vi "3-1.vi"() -> ()   [LabVIEW 2022 SP3, in "AoC22.lvlib"]
uses:
  AoC22.lvlib
  5f5b93ce-2920-4ca0-a169-f55fba87441a.vi
  <vilib>/IlluminatedG/lv-stream/Stream.lvlib
panel:
  out "sum":i32
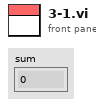
[diagram p1: front panel]
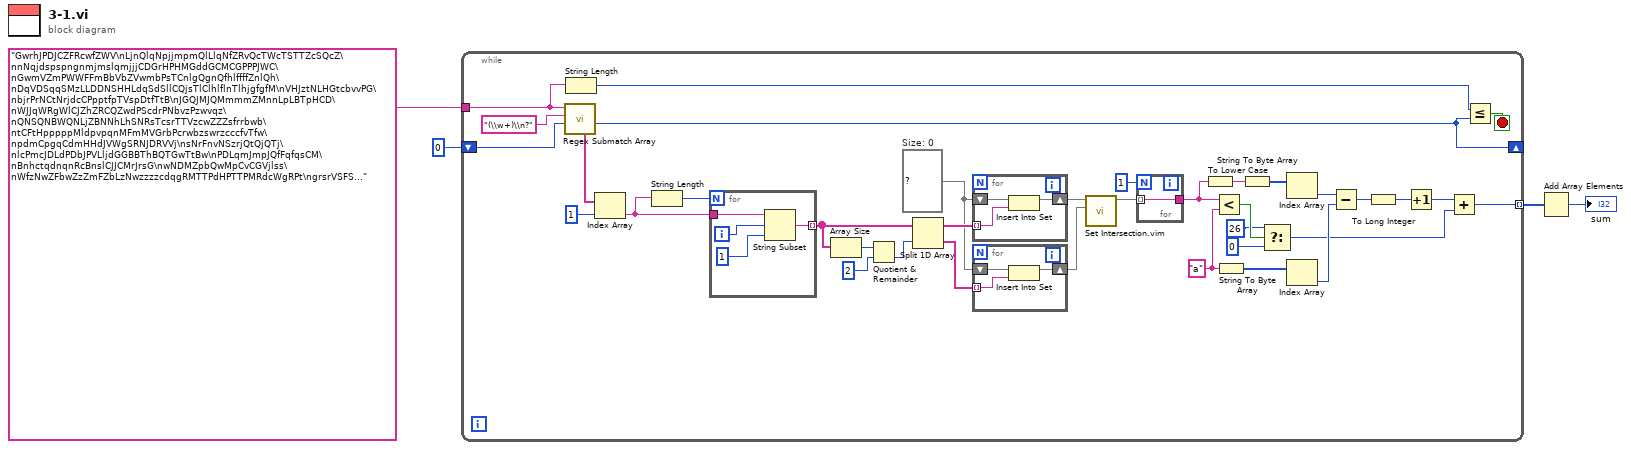
[diagram p0: block diagram]
diagram:
  n1 = while {
    tunnel: "GwrhJPDJCZFRcwfZWV\nLjnQlqNpjjmpmQlLlqNfZRvQcTWcTSTTZcSQcZ\nnNqjdspspngnmjmslqmjjjCDGrHPHMGddGCMCGPPPJWC\nGwmVZmPWWFFmBbVbZVwmbPsTCnlgQgnQfhlffffZnlQh\nDqVDSqqSMzLLDDNSHHLdqSdSllCQjsTlClhlflnTlhjgfgfM\nVHJztNLHGtcbvvPG\nbjrPrNCtNrjdcCPpptfpTVspDtfTtB\nJGQJMJQMmmmZMnnLpLBTpHCD\nWJJqWRgWlCJZhZRCQZwdPScdrPNbvzPzwvqz\nQNSQNBWQNLjZBNNhLhSNRsTcsrTTVzcwZZZsfrrbwb\ntCFtHpppppMldpvpqnMFmMVGrbPcrwbzswrzcccfvTfw\npdmCpgqCdmHHdJVWgSRNJDRVVj\nsNrFnvNSzrjQtQjQTj\nlcPmcJDLdPDbJPVLljdGGBBThBQTGwTtBw\nPDLqmJmpJQfFqfqsCM\nBnhctqdnqnRcBnslCJJCMrJrsG\nwNDMZpbQwMpCvCGVjlss\nWfzNwZFbwZzZmFZbLzNwzzzzcdqgRMTTPdHPTTPMRdcWgRPt\ngrsrVSFS..." -> [w8]
    shift-right: [w6] -> _
    shift-left: 0 -> [w39]
    tunnel: [w12] -> w2 mode=indexing
    stop <- w5 stop-if-true
    w25 = "a" ("y")
    w31 = set{string} {}  # Size: 0
    n2 = call <vilib>:"Regex Submatch Array.vi"("offset (0)"=w39, "regular expression"="(\\w+)\\n?", "string"=w8) -> ("offset past match"=w6:i32, "matches"=w38:string[])  [unwired: 6 in, 1 out]
    n3 = String Length(string=w8) -> (length=w7:i32)
    n4 = Index Array(array=w38, index=1) -> (element=w11:string)
    n5 = String Length(string=w11) -> (length=w10:i32)
    n6 = for {
      N: w10 -> [_]
      tunnel: w11 -> [w51]
      tunnel: [w48] -> w34 mode=indexing
      i -> [w50]
      n7 = String Subset(string=w51, offset (0)=w50, length (rest)=1 ("length (rest)")) -> (substring=w48:string)
    }
    n8 = Array Size(array=w34) -> (size(s)=w36:i32)
    n9 = Quotient & Remainder(x=w36, y=2) -> (floor(x/y)=w33:i32)  [unwired: 1 out]
    n10 = Split 1D Array(array=w34, index=w33) -> (first subarray=w32:string[], second subarray=w30:string[])
    n11 = for {
      tunnel: w32 -> [w46] mode=indexing
      shift-right: [w45] -> w29
      shift-left: w31 -> [w47]
      n12 = Insert Into Set(10:w46, 11:w47) -> (3:w45:set{string})  [unwired: 1 out]
    }
    n13 = for {
      tunnel: w30 -> [w43] mode=indexing
      shift-right: [w42] -> w28
      shift-left: w31 -> [w44]
      n14 = Insert Into Set(10:w43, 11:w44) -> (3:w42:set{string})  [unwired: 1 out]
    }
    n15 = call "Set Intersection.vim"("set 2"=w28, "set 1"=w29) -> ("intersection"=w27:set{string})  [unwired: 9 in]
    n16 = for {
      N: 1 -> [_]
      tunnel: w27 -> [w41] mode=indexing
      tunnel: [w41] -> w9
    }
    n17 = To Lower Case(string=w9) -> (all lower case string=w24:string)
    n18 = Less?(x=w9, y=w25) -> (x < y?=w19:bool)
    n19 = String To Byte Array(string=w25) -> (unsigned byte array=w22:u8[])
    n20 = String To Byte Array(string=w24) -> (unsigned byte array=w23:u8[])
    n21 = Select(t=26, s=w19, f=0) -> (s? t:f=w15:i32)
    n22 = Index Array(array=w23) -> (element=w21:u8)  [unwired: 1 in]
    n23 = Index Array(array=w22) -> (element=w20:u8)  [unwired: 1 in]
    n24 = Subtract(x=w21, y=w20) -> (x-y=w14:u8)
    n25 = To Long Integer(number=w14) -> (32bit integer=w13:i32)
    n26 = Increment(x=w13) -> (x+1=w16:i32)
    n27 = Add(x=w16, y=w15) -> (x+y=w12:i32)
    n28 = Less Or Equal?(x=w7, y=w6) -> (x <= y?=w5:bool)
  }
  n29 = Add Array Elements(numeric array=w2) -> (sum=→"sum":i32)
